vi "T7 Stream Config KAG-v2.vi"(0 "IP Configuration":T2={"Connection ID In"=refnum, "Connection ID Out"=refnum, "Device IP"="192.168.126.147", "Port"=502}, 5 "Stream Configuration":T3={"Scan Rate (Hz)"=1000.0, "Samples Per Packet"=512, "Resolution Index"=0, "Buffer Size (bytes)"=32768, "NumScans"=1500, "Read Timeout (ms)"=5000, "Scan Table"=[{"Channel"=0, "BipGain"=0, "Input Config"="Single-Ended"}, {"Channel"=1, "BipGain"=0, "Input Config"="Single-Ended"}, {"Channel"=2, "BipGain"=0, "Input Config"="Single-Ended"}, {"Channel"=3, "BipGain"=0, "Input Config"="Single-Ended"}]} {"Samples Per Packet" max=512 step=1; "Buffer Size (bytes)" max=32768 step=1; "Resolution Index" max=8 step=1; "Scan Rate (Hz)" max=100000; "Scan Table"."BipGain" items=["x1", "x10", "x100", "x1000"]; "Scan Table"."Channel" step=1}, 10 "STREAM Registers":T4(array[cluster])=[{"Register Num"=4990, "Register Name"="STREAM_ENABLE", "DataType"="UINT32", "Write Val"=0.0}, {"Register Num"=4002, "Register Name"="STREAM_SCANRATE_HZ", "DataType"="FLOAT32", "Write Val"=1000.0}, {"Register Num"=4004, "Register Name"="STREAM_NUM_ADDRESSES", "DataType"="UINT32", "Write Val"=4.0}, {"Register Num"=4006, "Register Name"="STREAM_SAMPLES_PER_PACKET", "DataType"="UINT32", "Write Val"=25000.0}, {"Register Num"=4008, "Register Name"="STREAM_SETTLING_US", "DataType"="FLOAT32", "Write Val"=0.0}, {"Register Num"=4010, "Register Name"="STREAM_RESOLUTION_INDEX", "DataType"="UINT32", "Write Val"=0.0}, {"Register Num"=4012, "Register Name"="STREAM_BUFFER_SIZE_BYTES", "DataType"="UINT32", "Write Val"=20000.0}, {"Register Num"=4014, "Register Name"="STREAM_OPTIONS", "DataType"="UINT32", "Write Val"=0.0}, {"Register Num"=4016, "Register Name"="STREAM_AUTO_TARGET", "DataType"="UINT32", "Write Val"=0.0}, {"Register Num"=4018, "Register Name"="STREAM_DATATYPE", "DataType"="UINT32", "Write Val"=0.0}, {"Register Num"=4020, "Register Name"="STREAM_NUM_SCANS", "DataType"="UINT32", "Write Val"=1500.0}, {"Register Num"=4022, "Register Name"="STREAM_EXTERNAL_CLOCK_DIVISOR", "DataType"="UINT32", "Write Val"=0.0}, {"Register Num"=4100, "Register Name"="STREAM_SCANLIST_ADDRESS#(0:127)", "DataType"="UINT32", "Write Val"=0.0}, {"Register Num"=4102, "Register Name"="STREAM_SCANLIST_ADDRESS#(0:127)", "DataType"="UINT32", "Write Val"=2.0}, {"Register Num"=4104, "Register Name"="STREAM_SCANLIST_ADDRESS#(0:127)", "DataType"="UINT32", "Write Val"=4.0}, {"Register Num"=4106, "Register Name"="STREAM_SCANLIST_ADDRESS#(0:127)", "DataType"="UINT32", "Write Val"=5.0}, {"Register Num"=41000, "Register Name"="AIN#(0:254)_NEGATIVE_CH", "DataType"="UINT16", "Write Val"=199.0}, {"Register Num"=41002, "Register Name"="AIN#(0:254)_NEGATIVE_CH", "DataType"="UINT16", "Write Val"=3.0}, {"Register Num"=41004, "Register Name"="AIN#(0:254)_NEGATIVE_CH", "DataType"="UINT16", "Write Val"=199.0}], 11 "error in":errorcluster) -> (6 "Strm Config Out":T3={"Scan Rate (Hz)"=1000.0, "Samples Per Packet"=512, "Resolution Index"=0, "Buffer Size (bytes)"=32768, "NumScans"=1500, "Read Timeout (ms)"=5000, "Scan Table"=[{"Channel"=0, "BipGain"=0, "Input Config"="Single-Ended"}, {"Channel"=1, "BipGain"=0, "Input Config"="Single-Ended"}, {"Channel"=2, "BipGain"=0, "Input Config"="Single-Ended"}, {"Channel"=3, "BipGain"=0, "Input Config"="Single-Ended"}]} {"Samples Per Packet" max=512 step=1; "Buffer Size (bytes)" max=32768 step=1; "Resolution Index" max=8 step=1; "Scan Rate (Hz)" max=100000; "Scan Table"."BipGain" items=["x1", "x10", "x100", "x1000"]; "Scan Table"."Channel" step=1}, 15 "error out":errorcluster)   [LabVIEW 2015]
doc: "Write Stream Configuration LabJack Registers via MODBUS. There are a set of registers which comprise the stream configuration registers, and these are written with control values for Scan Rate, NumScans, Resolution, etc. Also, the Scan Table is used to build a Scan List of Stream Configuration Registers which point to streamable AI Channels."
uses:
  T7 Stream Config KAG.ctl
  T7 IP Config KAG.ctl
  T7 Secondary Configs KAG.ctl
  T7Examples/MODBUS/T7MOD_Write_UINT16_Register.vi
  T7Examples/MODBUS/T7MOD_Write_FLOAT32_Register.vi
panel:
  in  "Secondary Stream Configurations":T1={"Settling Delay (*5 us)"=0.0, "Clock Source"=0, "Auto Target"=1} {"Auto Target" max=5000 step=1; "Clock Source" max=2 step=2; "Settling Delay (*5 us)" max=255 step=1}
  in  "Tab Control":enum32{"Stream Registers", "Stream Config Out"}(tab)
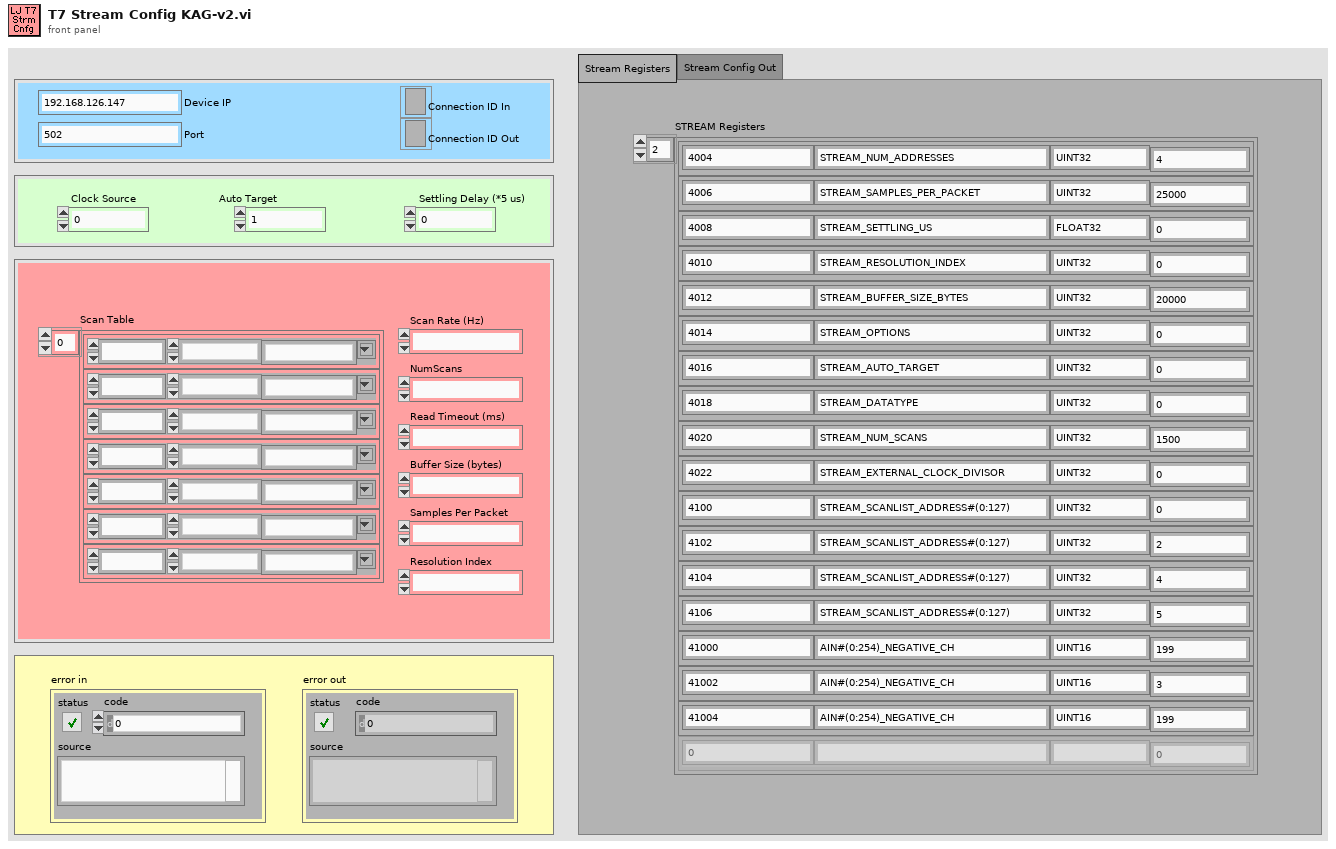
[diagram p1: front panel]
types:
  T1 = typedef "T7 Secondary Configs KAG.ctl" = cluster{"Settling Delay (*5 us)":sgl, "Clock Source":u32, "Auto Target":u32}
  T2 = typedef "T7 IP Config KAG.ctl" = cluster{"Connection ID In":refnum<k5>, "Connection ID Out":refnum<k5>, "Device IP":string, "Port":i32}
  T3 = typedef "T7 Stream Config KAG.ctl" = cluster{"Scan Rate (Hz)":sgl, "Samples Per Packet":u32, "Resolution Index":u32, "Buffer Size (bytes)":u32, "NumScans":u32, "Read Timeout (ms)":u32, "Scan Table":cluster{"Channel":u32, "BipGain":u32, "Input Config":string}[]}
  T4 = cluster{"Register Num":i32, "Register Name":string, "DataType":string, "Write Val":dbl}[]
  T5 = cluster{"Channel":u32, "BipGain":u32, "Input Config":string}[]
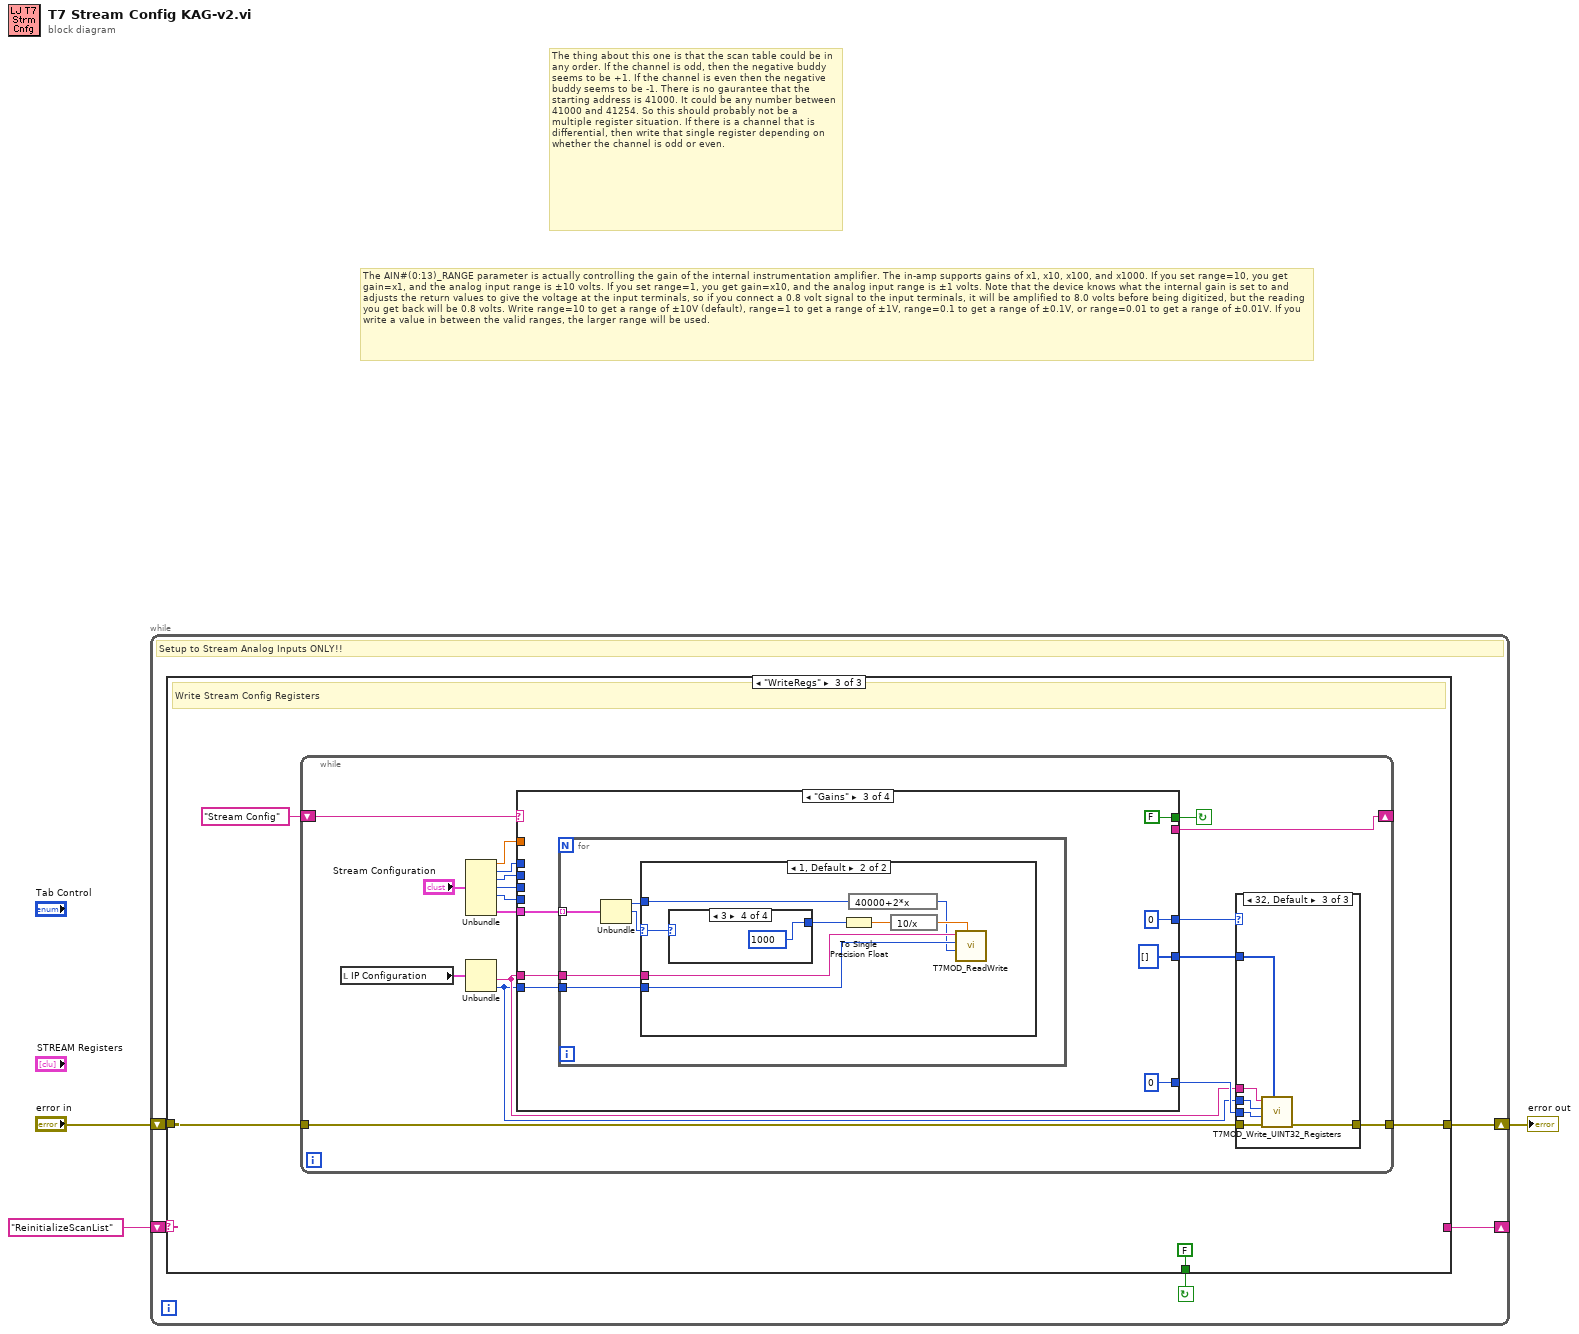
[diagram p0: block diagram]
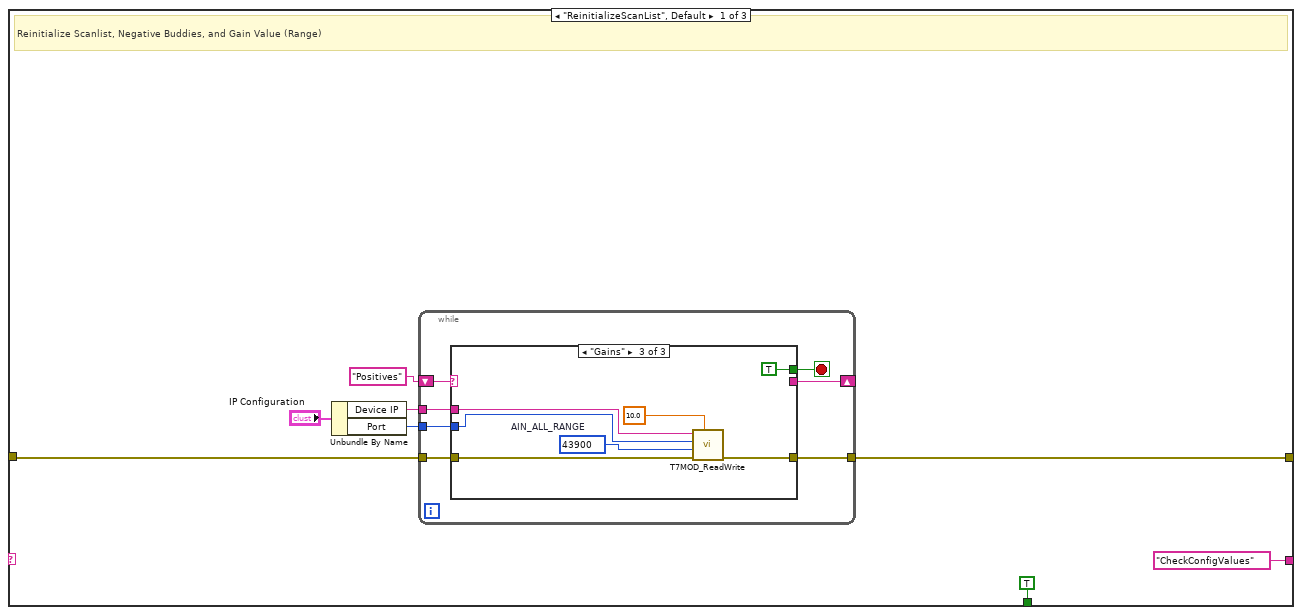
[diagram p2: hidden frame]
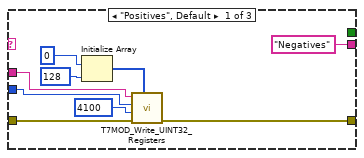
[diagram p3: hidden frame]
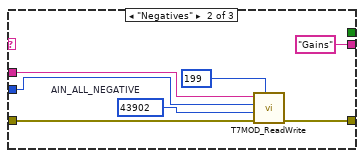
[diagram p4: hidden frame]
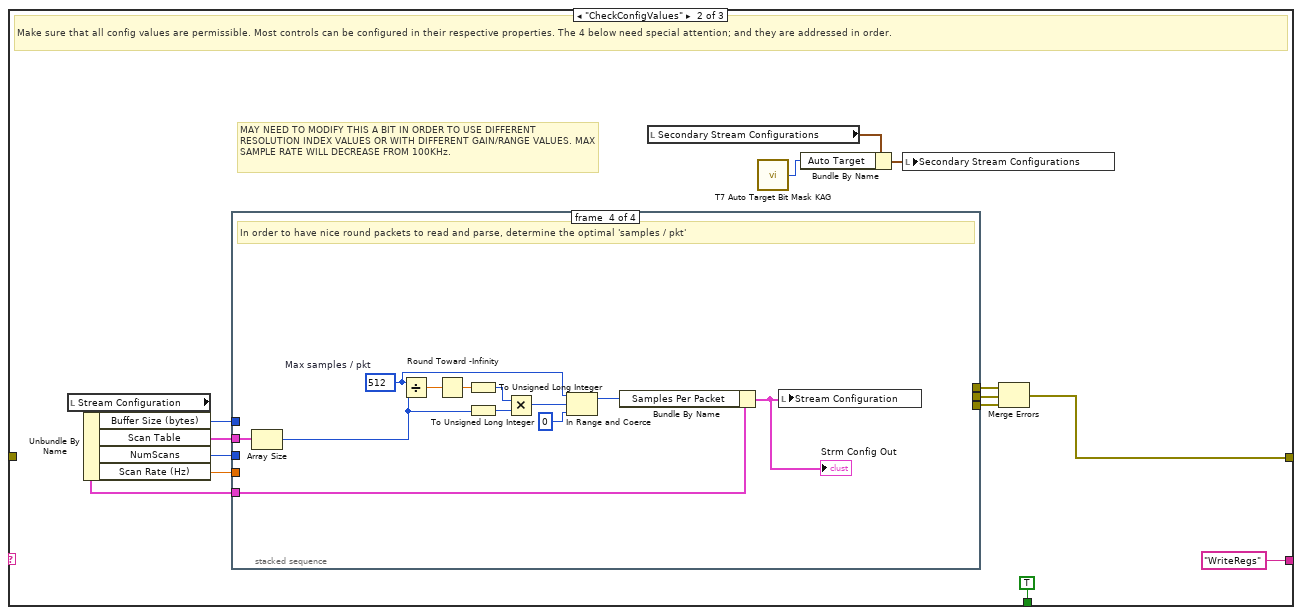
[diagram p5: hidden frame]
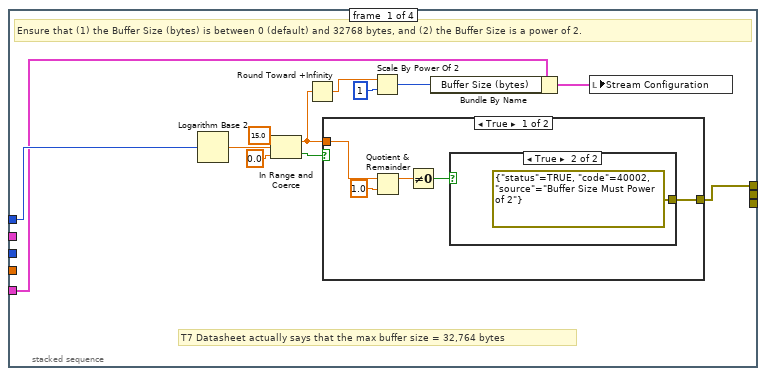
[diagram p6: hidden frame]
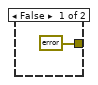
[diagram p7: hidden frame]
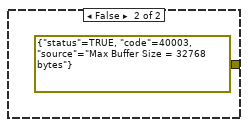
[diagram p8: hidden frame]
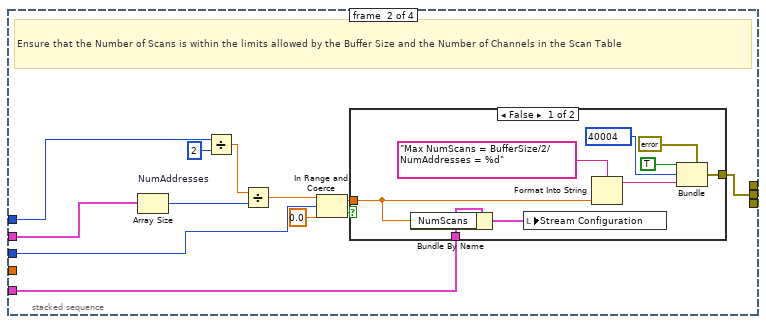
[diagram p9: hidden frame]
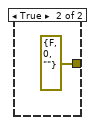
[diagram p10: hidden frame]
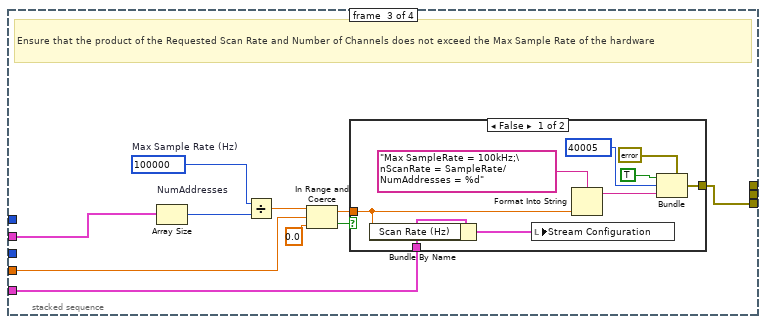
[diagram p11: hidden frame]
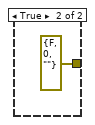
[diagram p12: hidden frame]
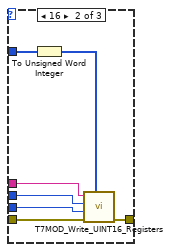
[diagram p14: hidden frame]
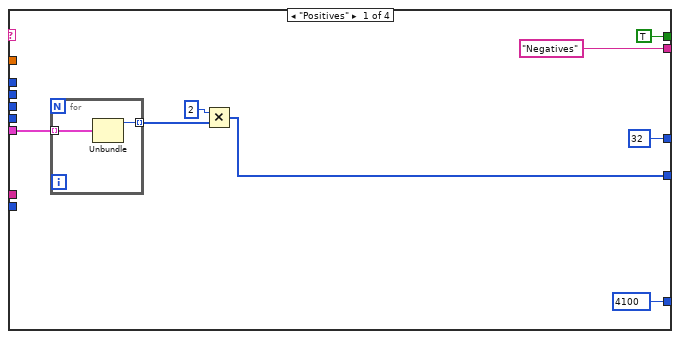
[diagram p15: hidden frame]
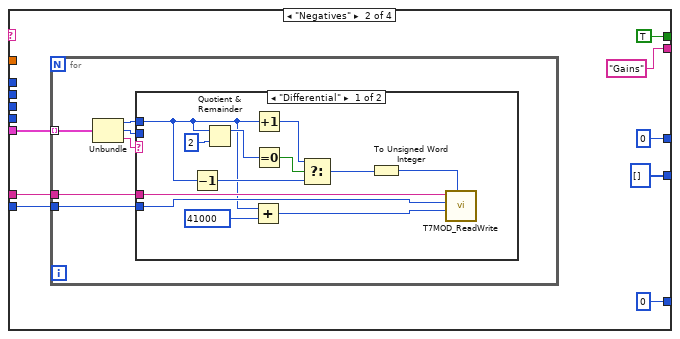
[diagram p16: hidden frame]
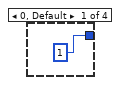
[diagram p19: hidden frame]
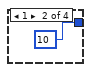
[diagram p20: hidden frame]
diagram:
  # "The AIN#(0:13)_RANGE parameter is actually controlling the gain of the internal instrumentation amplifier. The in-amp supports gains of x1, x10, x100, and x1000. If you set range=10, you get gain=x1, and the analog input range is ±10 volts. If you set range=1, you get gain=x10, and the analog input range is ±1 volts. Note that the device knows what the internal gain is set to and adjusts the return values to give the voltage at the input terminals, so if you connect a 0.8 volt signal to the input terminals, it will be amplified to 8.0 volts before being digitized, but the reading you get back will be 0.8 volts. Write range=10 to get a range of ±10V (default), range=1 to get a range of ±1V, range=0.1 to get a range of ±0.1V, or range=0.01 to get a range of ±0.01V. If you write a value in between the valid ranges, the larger range will be used."
  # "The thing about this one is that the scan table could be in any order. If the channel is odd, then the negative buddy seems to be +1. If the channel is even then the negative buddy seems to be -1. There is no gaurantee that the starting address is 41000. It could be any number between 41000 and 41254. So this should probably not be a multiple register situation. If there is a channel that is differential, then write that single register depending on whether the channel is odd or even."
  n1 = while {
    shift-right: [w6] -> _
    shift-left: "ReinitializeScanList" -> [w8]
    shift-right: [w4] -> w1
    shift-left: "error in" -> [w5]
    stop <- w7 continue-if-true
    # "Setup to Stream Analog Inputs ONLY!!"
    n2 = case shown="\"WriteRegs\"" w8 {
      tunnel: [TRUE TRUE FALSE] -> w7
      tunnel: ["CheckConfigValues" "WriteRegs" _] -> w6
      tunnel: w5 -> [w12 _ w136]
      tunnel: [w11 w55 w135] -> w4
      frame "ReinitializeScanList", Default {
        # "Reinitialize Scanlist, Negative Buddies, and Gain Value (Range)"
        n3 = Unbundle By Name("IP Configuration") -> ("Device IP"=w10:string, "Port"=w9:i32)
        n4 = while {
          shift-right: [w22] -> _
          shift-left: "Positives" -> [w23]
          tunnel: w12 -> [w20]
          tunnel: [w19] -> w11
          tunnel: w10 -> [w18]
          tunnel: w9 -> [w17]
          stop <- w21 stop-if-true
          n5 = case shown="\"Gains\"" w23 {
            tunnel: ["Negatives" "Gains" _] -> w22
            tunnel: [_ _ TRUE] -> w21
            tunnel: w20 -> [w27 w36 w43]
            tunnel: [w26 w35 w42] -> w19
            tunnel: w18 -> [w25 w34 w41]
            tunnel: w17 -> [w24 w33 w40]
            frame "Positives", Default {
              n6 = Initialize Array(u32 0 ("UINT32 to Write"), 128) -> (w29:u32[])
              n7 = call "T7MOD_Write_UINT32_Registers.vi"("UINT32 to Write"=w29, "error in"=w27, "Starting Address"=4100, "Remote Port"=w24, "Remote IP Address"=w25) -> ("error out"=w26:errorcluster)  [unwired: 5 in, 1 out]
            }
            frame "Negatives" {
              w37 = 43902  # AIN_ALL_NEGATIVE
              n8 = call-poly "T7MOD_ReadWrite.vi"("UINT16 to Write"=u16 199 ("UINT32 to Write"), "error in"=w36, "LabJack UINT16 Register"=w37, "Remote Port"=w33, "Remote IP Address"=w34) -> ("error out"=w35:errorcluster)  [unwired: 5 in, 1 out]
            }
            frame "Gains" {
              w46 = 43900  # AIN_ALL_RANGE
              n9 = call-poly "T7MOD_ReadWrite.vi"("FLOAT32 to Write"=sgl 10.0, "error in"=w43, "LabJack FLOAT32 Register"=w46, "Remote Port"=w40, "Remote IP Address"=w41) -> ("error out"=w42:errorcluster)  [unwired: 5 in, 1 out]
            }
          }
        }
      }
      frame "CheckConfigValues" {
        # "MAY NEED TO MODIFY THIS A BIT IN ORDER TO USE DIFFERENT RESOLUTION INDEX VALUES OR WITH DIFFERENT GAIN/RANGE VALUES. MAX SAMPLE RATE WILL DECREASE FROM 100KHz."
        # "Make sure that all config values are permissible. Most controls can be configured in their respective properties. The 4 below need special attention; and they are addressed in order."
        n10 = local read "Stream Configuration"() -> (w48:T3)
        n11 = Unbundle By Name(w48) -> ("Buffer Size (bytes)"=w51:u32, "Scan Table"=w52:T5, "NumScans"=w53:u32, "Scan Rate (Hz)"=w50:sgl)
        n12 = stacked-sequence {
          tunnel: [w64 _ _ _] -> w58
          tunnel: [_ w85 _ _] -> w57
          tunnel: [_ _ w106 _] -> w56
          tunnel: w48 -> [w61 w84 w103 w130]
          tunnel: w53 -> [_ w83 _ _]
          tunnel: w52 -> [_ w82 w105 w132]
          tunnel: w51 -> [w62 w81 _ _]
          tunnel: w50 -> [_ _ w104 _]
          frame #0 {
            # "T7 Datasheet actually says that the max buffer size = 32,764 bytes"
            # "Ensure that (1) the Buffer Size (bytes) is between 0 (default) and 32768 bytes, and (2) the Buffer Size is a power of 2."
            n13 = Logarithm Base 2(1:w62) -> (0:w71:dbl)
            n14 = In Range and Coerce(upper limit=15.0 ("y"), x=w71, lower limit=0.0) -> (coerced(x)=w65:dbl, In Range?=w69:bool)
            n15 = Round Toward +Infinity(x=w65) -> (ceil(x): smallest int >= x=w67:dbl)
            n16 = case shown="True" w69 {
              tunnel: [w75 errorcluster {"status"=TRUE, "code"=40003, "source"="Max Buffer Size = 32768 bytes"} ("error constant")] -> w64
              tunnel: w65 -> [w73 _]
              frame True {
                n17 = Quotient & Remainder(x=w73, y=1.0) -> (x-y*floor(x/y)=w76:dbl)  [unwired: 1 out]
                n18 = Not Equal To 0?(x=w76) -> (x != 0?=w74:bool)
                n19 = case shown="True" w74 {
                  tunnel: [errorcluster {"status"=FALSE, "code"=0, "source"=""} ("error constant") errorcluster {"status"=TRUE, "code"=40002, "source"="Buffer Size Must Power of 2"} ("error constant")] -> w75
                  frame False {
                  }
                  frame True {
                  }
                }
              }
              frame False {
              }
            }
            n20 = Scale By Power Of 2(n=w67, x=u32 1) -> (x*2^n=w68:u32)
            n21 = Bundle By Name(cluster=w61, "Buffer Size (bytes)"=w68) -> (w63:T3)
            n22 = local write "Stream Configuration"(w63) -> ()
          }
          frame #1 {
            # "Ensure that the Number of Scans is within the limits allowed by the Buffer Size and the Number of Channels in the Scan Table"
            n23 = Array Size "NumAddresses"(array=w82) -> (size(s)=w92:i32)
            n24 = Divide(x=w81, y=u32 2) -> (x/y=w91:dbl)
            n25 = Divide(x=w91, y=w92) -> (x/y=w89:dbl)
            n26 = In Range and Coerce(upper limit=w89, x=w83, lower limit=0.0) -> (coerced(x)=w87:dbl, In Range?=w86:bool)
            n27 = case shown="False" w86 {
              tunnel: w87 -> [w95 _]
              tunnel: [w96 errorcluster {"status"=FALSE, "code"=0, "source"=""} ("error constant")] -> w85
              tunnel: w84 -> [w93 _]
              frame False {
                n28 = Bundle By Name(cluster=w93, "NumScans"=w95) -> (w94:T3)
                n29 = local write "Stream Configuration"(w94) -> ()
                n30 = Format Into String(format string="Max NumScans = BufferSize/2/NumAddresses = %d" ("initial string"), w95) -> (resulting string=w97:string)  [unwired: 2 in, 1 out]
                n31 = Bundle(cluster=errorcluster {"status"=FALSE, "code"=0, "source"=""} ("error constant"), "status"=TRUE, "code"=40004, "source"=w97) -> (w96:errorcluster)
              }
              frame True {
              }
            }
          }
          frame #2 {
            w111 = 100000  # Max Sample Rate (Hz)
            # "Ensure that the product of the Requested Scan Rate and Number of Channels does not exceed the Max Sample Rate of the hardware"
            n32 = Array Size "NumAddresses"(array=w105) -> (size(s)=w112:i32)
            n33 = Divide(x=w111, y=w112) -> (x/y=w110:dbl)
            n34 = In Range and Coerce(upper limit=w110, x=w104, lower limit=0.0) -> (coerced(x)=w107:dbl, In Range?=w108:bool)
            n35 = case shown="False" w108 {
              tunnel: w107 -> [w115 _]
              tunnel: [w116 errorcluster {"status"=FALSE, "code"=0, "source"=""} ("error constant")] -> w106
              tunnel: w103 -> [w113 _]
              frame False {
                n36 = Bundle By Name(cluster=w113, "Scan Rate (Hz)"=w115) -> (w114:T3)
                n37 = local write "Stream Configuration"(w114) -> ()
                n38 = Format Into String(format string="Max SampleRate = 100kHz;\nScanRate = SampleRate/NumAddresses = %d" ("initial string"), w115) -> (resulting string=w117:string)  [unwired: 2 in, 1 out]
                n39 = Bundle(cluster=errorcluster {"status"=FALSE, "code"=0, "source"=""} ("error constant"), "status"=TRUE, "code"=40005, "source"=w117) -> (w116:errorcluster)
              }
              frame True {
              }
            }
          }
          frame #3 {
            w125 = 512  # Max samples / pkt
            # "In order to have nice round packets to read and parse, determine the optimal 'samples / pkt'"
            n40 = Array Size(array=w132) -> (size(s)=w131:i32)
            n41 = Divide(x=w125, y=w131) -> (x/y=w134:dbl)
            n42 = Round Toward -Infinity(1:w134) -> (0:w133:dbl)
            n43 = To Unsigned Long Integer(number=w133) -> (unsigned 32bit integer=w129:u32)
            n44 = To Unsigned Long Integer(number=w131) -> (unsigned 32bit integer=w128:u32)
            n45 = Multiply(x=w129, y=w128) -> (x*y=w127:u32)
            n46 = In Range and Coerce(upper limit=w125, x=w127, lower limit=u32 0) -> (coerced(x)=w124:u32)  [unwired: 1 out]
            n47 = Bundle By Name(cluster=w130, "Samples Per Packet"=w124) -> (w123:T3)
            "Strm Config Out" <- w123
            n48 = local write "Stream Configuration"(w123) -> ()
          }
        }
        n49 = local read "Secondary Stream Configurations"() -> (w47:T1)
        n50 = call "T7 Auto Target Bit Mask KAG.vi"() -> ("Auto Target"=w54:u32)  [unwired: 1 in]
        n51 = Bundle By Name(cluster=w47, "Auto Target"=w54) -> (w49:T1)
        n52 = local write "Secondary Stream Configurations"(w49) -> ()
        n53 = Merge Errors(w58, w57, w56) -> (w55:errorcluster)
      }
      frame "WriteRegs" {
        # "Write Stream Config Registers"
        n54 = while {
          shift-right: [w141] -> _
          shift-left: "Stream Config" -> [w146]
          tunnel: w136 -> [w144]
          tunnel: [w143] -> w135
          stop <- w142 continue-if-true
          n55 = local read "IP Configuration"() -> (w154:T2)
          n56 = Unbundle("Stream Configuration") -> ("Scan Rate (Hz)"=w151:sgl, "Samples Per Packet"=w150:u32, "Resolution Index"=w149:u32, "Buffer Size (bytes)"=w148:u32, "NumScans"=w147:u32, "Scan Table"=w152:T5)  [unwired: 1 out]
          n57 = Unbundle(w154) -> ("Device IP"=w140:string, "Port"=w139:i32)  [unwired: 2 out]
          n58 = case shown="\"Gains\"" w146 {
            tunnel: [4100 ("Starting Address") 0 ("Starting Address") 0 ("Starting Address") 4002 ("Starting Address")] -> w156
            tunnel: [w175 u32[] [] u32[] [] w240] -> w155
            tunnel: w152 -> [w174 w188 w213 w234]
            tunnel: w151 -> [_ _ _ w239]
            tunnel: w150 -> [_ _ _ w238]
            tunnel: w149 -> [_ _ _ w237]
            tunnel: w148 -> [_ _ _ w236]
            tunnel: w147 -> [_ _ _ w235]
            tunnel: [32 0 0 32] -> w145
            tunnel: [TRUE TRUE FALSE TRUE] -> w142
            tunnel: ["Negatives" "Gains" _ "Positives"] -> w141
            tunnel: w140 -> [_ w185 w210 _]
            tunnel: w139 -> [_ w184 w209 _]
            frame "Positives" {
              n59 = for {
                tunnel: w174 -> [w180] mode=indexing
                tunnel: [w179] -> w177 mode=indexing
                n60 = Unbundle(w180) -> ("Channel"=w179:u32)  [unwired: 2 out]
              }
              n61 = Multiply(x=u32 2, y=w177) -> (x*y=w175:u32[])
            }
            frame "Negatives" {
              n62 = for {
                tunnel: w188 -> [w194] mode=indexing
                tunnel: w185 -> [w191]
                tunnel: w184 -> [w190]
                n63 = Unbundle(w194) -> ("Channel"=w192:u32, "BipGain"=w189:u32, "Input Config"=w193:string)
                n64 = case shown="\"Differential\"" w193 {
                  tunnel: w192 -> [w195 _]
                  tunnel: w191 -> [w202 _]
                  tunnel: w190 -> [w201 _]
                  tunnel: w189 -> [_ _]
                  frame "Differential" {
                    n65 = Decrement(x=w195) -> (x-1=w204:u32)
                    n66 = Quotient & Remainder(x=w195, y=u32 2) -> (x-y*floor(x/y)=w197:u32)  [unwired: 1 out]
                    n67 = Add(x=w195, y=41000 ("Starting Address")) -> (x+y=w203:u32)
                    n68 = Increment(x=w195) -> (x+1=w205:u32)
                    n69 = Equal To 0?(x=w197) -> (x = 0?=w206:bool)
                    n70 = Select(t=w205, s=w206, f=w204) -> (s? t:f=w200:u32)
                    n71 = To Unsigned Word Integer(number=w200) -> (unsigned 16bit integer=w199:u16)
                    n72 = call-poly "T7MOD_ReadWrite.vi"("UINT16 to Write"=w199, "LabJack UINT16 Register"=w203, "Remote Port"=w201, "Remote IP Address"=w202) -> ()  [unwired: 6 in, 2 out]
                  }
                  frame "Single-Ended", Default {
                  }
                }
              }
            }
            frame "Gains" {
              n73 = for {
                tunnel: w213 -> [w218] mode=indexing
                tunnel: w210 -> [w217]
                tunnel: w209 -> [w216]
                n74 = Unbundle(w218) -> ("Channel"=w214:u32, "BipGain"=w215:u32)  [unwired: 1 out]
                n75 = case shown="1, Default" w215 {
                  selector: w215 -> [_ w220]
                  tunnel: w214 -> [_ w226]
                  tunnel: w217 -> [_ w224]
                  tunnel: w216 -> [_ w223]
                  frame 0 {
                  }
                  frame 1, Default {
                    n76 = case shown="3" w220 {
                      tunnel: [1 10 100 1000] -> w219
                      frame 0, Default {
                      }
                      frame 1 {
                      }
                      frame 2 {
                      }
                      frame 3 {
                      }
                    }
                    n77 = To Single Precision Float(number=w219) -> (single precision float=w225:sgl)
                    n78 = expression code="40000+2*x"(w226) -> (w221:u32)
                    n79 = expression code="10/x"(w225) -> (w222:sgl)
                    n80 = call-poly "T7MOD_ReadWrite.vi"("FLOAT32 to Write"=w222, "LabJack FLOAT32 Register"=w221, "Remote Port"=w223, "Remote IP Address"=w224) -> ()  [unwired: 6 in, 2 out]
                  }
                }
              }
            }
            frame "Stream Config", Default {
              w242 = u32 0
              w252 = u32 0
              n81 = Array Size "Num Addresses"(array=w234) -> (size(s)=w250:i32)
              n82 = disable-structure shown="Enabled" {
                disable-tunnel: [w253 u32 0 ("NumScans")] -> w251
                disable-tunnel: w235 -> [w253 _]
                frame Disabled {
                }
                frame Enabled {
                }
              }
              n83 = To Unsigned Long Integer(number=w250) -> (unsigned 32bit integer=w244:u32)
              n84 = Unbundle("Secondary Stream Configurations") -> ("Settling Delay (*5 us)"=w248:sgl, "Clock Source"=w247:u32, "Auto Target"=w246:u32)
              n85 = Type Cast(type=w242, x=w239) -> (*(type *) &x=w245:u32)
              n86 = Type Cast(type=w242, x=w248) -> (*(type *) &x=w243:u32)
              n87 = Build Array(w245, w244, w238, w243, w237, w236, w247, w246, w252, w251, w252) -> (w240:u32[])
            }
          }
          n88 = case shown="32, Default" w145 {
            tunnel: w156 -> [_ w161 w170]
            tunnel: w155 -> [_ w164 w169]
            tunnel: w140 -> [_ w163 w168]
            tunnel: w139 -> [_ w162 w167]
            tunnel: w144 -> [w157 w160 w166]
            tunnel: [w157 w159 w165] -> w143
            frame 0 {
            }
            frame 16 {
              n89 = To Unsigned Word Integer(number=w164) -> (unsigned 16bit integer=w158:u16[])
              n90 = call "T7MOD_Write_UINT16_Registers.vi"("UINT16 to Write"=w158, "error in"=w160, "Starting Address"=w161, "Remote Port"=w162, "Remote IP Address"=w163) -> ("error out"=w159:errorcluster)  [unwired: 5 in, 1 out]
            }
            frame 32, Default {
              n91 = call "T7MOD_Write_UINT32_Registers.vi"("UINT32 to Write"=w169, "error in"=w166, "Starting Address"=w170, "Remote Port"=w167, "Remote IP Address"=w168) -> ("error out"=w165:errorcluster)  [unwired: 5 in, 1 out]
            }
          }
        }
      }
    }
  }
  "error out" <- w1
